vi "例4.7.vi"() -> ()   [LabVIEW 2018]
panel:
  in  "停止":bool
  out "乘积2":dbl
  out "乘积1":dbl
  in  "y":dbl
  in  "x":dbl
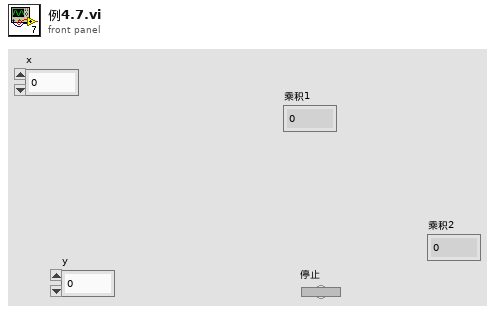
[diagram p1: front panel]
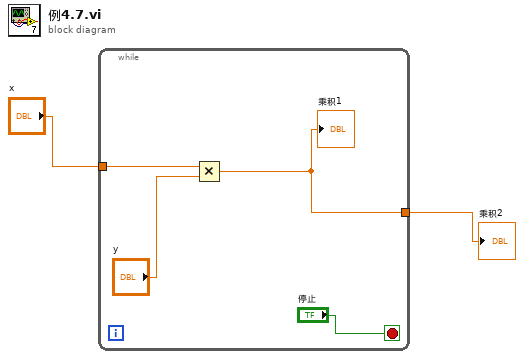
[diagram p0: block diagram]
diagram:
  n1 = while {
    tunnel: "x" -> [w5]
    tunnel: [w3] -> w1
    stop <- "停止" stop-if-true
    n2 = Multiply(x=w5, y="y") -> (x*y=w3:dbl)
    "乘积1" <- w3
  }
  "乘积2" <- w1
